vi "model_Path.vi"(10 "MODEL":string) -> (0 "TemplateB":path, 1 "TemplateA":path, 2 "TemplateC":path)   [LabVIEW 2013]
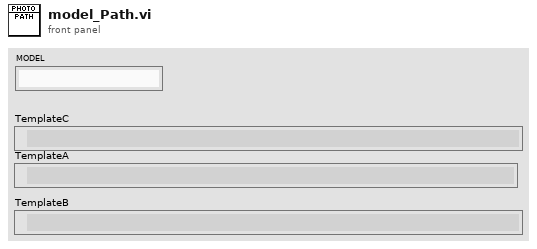
[diagram p1: front panel]
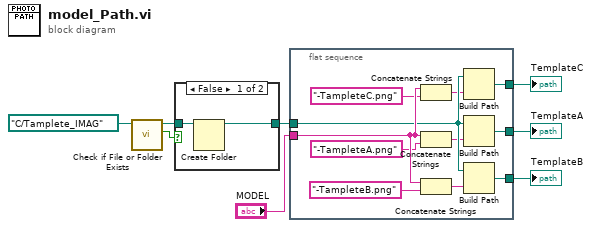
[diagram p0: block diagram]
diagram:
  n1 = call <vilib>:"Check if File or Folder Exists.vi"("path"=path "C:/Tamplete_IMAG" ("Template")) -> ("file or folder exists?"=w4:bool, "dup path"=w1:path)  [unwired: 8 in, 1 out]
  n2 = case shown="False" w4 {
    tunnel: [w9 w11] -> w2
    tunnel: w1 -> [w10 w11]
    frame False {
      n3 = Create Folder(path (use dialog)=w10) -> (created path=w9:path)  [unwired: 2 in, 2 out]
    }
    frame True {
    }
  }
  n4 = flat-sequence {
    tunnel: [w22] -> w8
    tunnel: "MODEL" -> [w21]
    tunnel: [w20] -> w6
    tunnel: [w19] -> w5
    tunnel: w2 -> [w18]
    frame #0 {
      n5 = Concatenate Strings(w21, "-TampleteC.png" ("string")) -> (w16:string)
      n6 = Concatenate Strings(w21, "-TampleteA.png" ("string")) -> (w14:string)
      n7 = Concatenate Strings(w21, "-TampleteB.png" ("string")) -> (w12:string)
      n8 = Build Path(base path=w18, name or relative path=w16) -> (appended path=w19:path)
      n9 = Build Path(base path=w18, name or relative path=w14) -> (appended path=w22:path)
      n10 = Build Path(base path=w18, name or relative path=w12) -> (appended path=w20:path)
    }
  }
  "TemplateA" <- w8
  "TemplateB" <- w6
  "TemplateC" <- w5
